vi "FT10_Log TDMS Values.vi"(8 "error in":errorcluster, 9 "Filename Cluster in":T1, 10 "Log Cluster in":T6, 11 "Log Loop Cluster in":T2={"tdms file out"=refnum, "t0"="", "Generator Serial Number in"="T1234567DX"}) -> (0 "error out":errorcluster, 3 "Log Loop Cluster out":T2={"tdms file out"=refnum, "t0"="", "Generator Serial Number in"="T1234567DX"})   [LabVIEW 2024]
doc: "Saves current and diff voltage to the TDMS file created when application started."
uses:
  Controls/Control_Log Cluster.ctl
  Controls/Control_Log Time.ctl
  Controls/Control_Log Waveform Cluster - Current.ctl
  Controls/Control_Log Analysis Cluster - Current.ctl
  Controls/Control_Log Activation Settings Cluster.ctl
  Controls/Control_Log Unitherm Load.ctl
  Controls/Control_Log Port.ctl
  Controls/Control_Log Mode.ctl
  Controls/Control_Log Power Level.ctl
  Controls/Control_Log Waveform Cluster - Diff Voltage.ctl
  Controls/Control_Log Analysis Cluster - Diff Voltage.ctl
  Controls/Control_Log Loop Cluster.ctl
  Controls/Control_Log TDMS Filename.ctl
  Controls/Control_Log t0.ctl
  Controls/Control_Serial Number.ctl
  Controls/Control_Log Filename Cluster.ctl
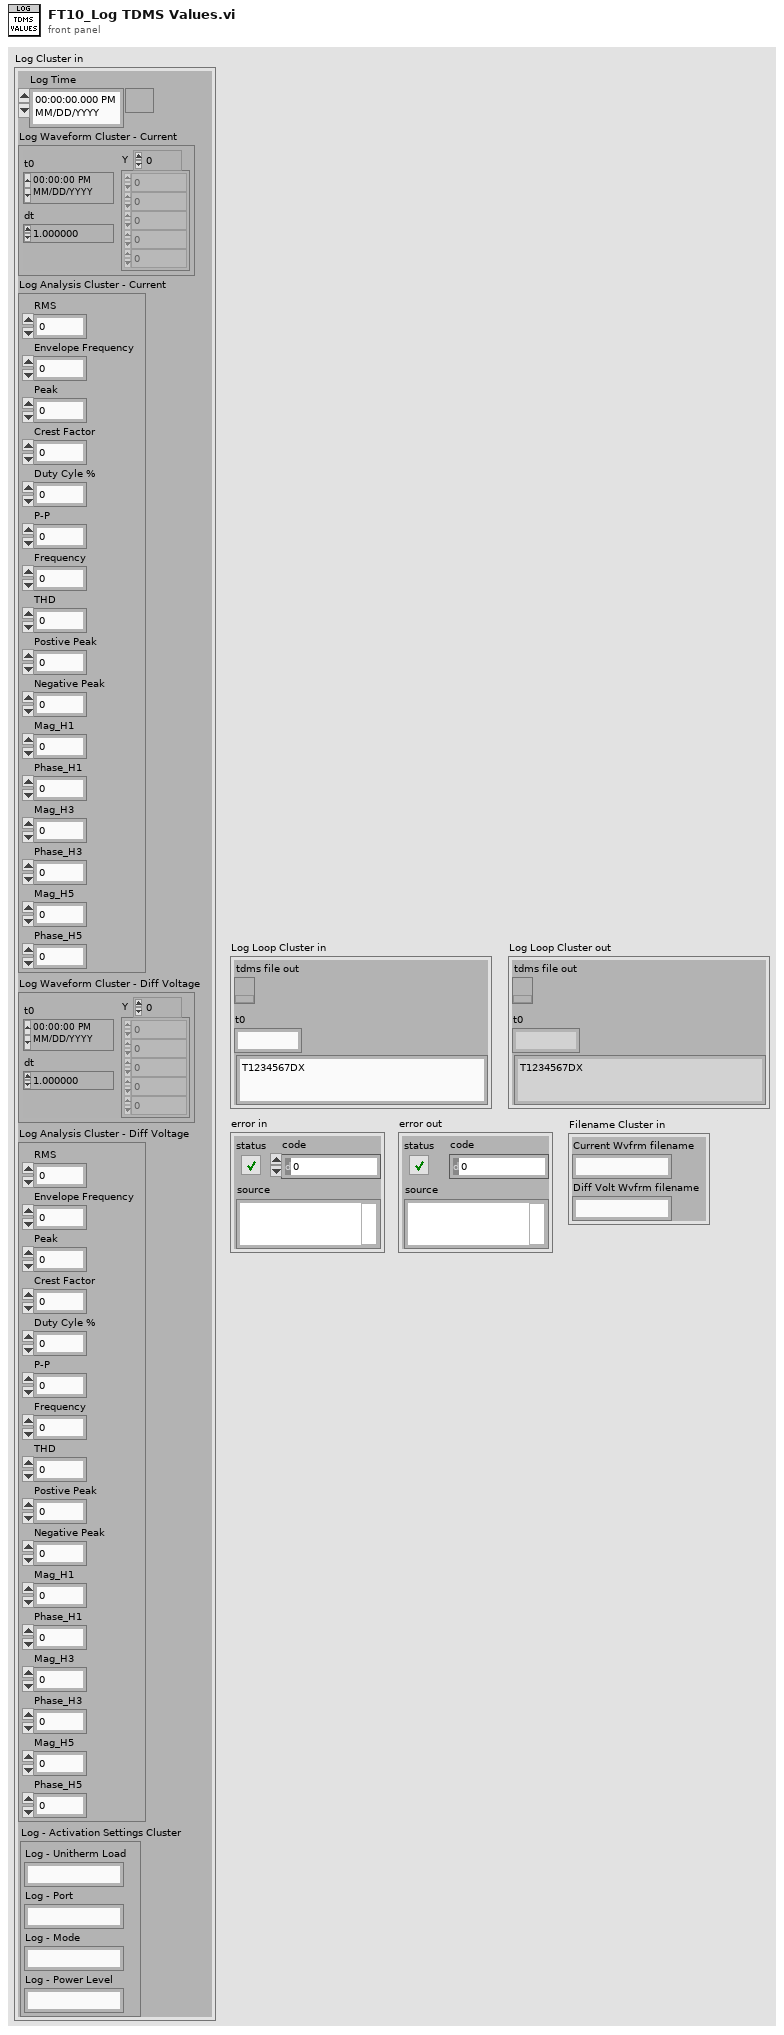
[diagram p1: front panel]
types:
  T1 = typedef "Control_Log Filename Cluster.ctl" = cluster{"Current Wvfrm filename":string, "Diff Volt Wvfrm filename":string}
  T2 = typedef "Control_Log Loop Cluster.ctl" = cluster{"tdms file out":T3, "t0":T4, "Generator Serial Number in":T5}
  T3 = typedef "Control_Log TDMS Filename.ctl" = refnum<k34>
  T4 = typedef "Control_Log t0.ctl" = string
  T5 = typedef "Control_Serial Number.ctl" = string
  T6 = typedef "Control_Log Cluster.ctl" = cluster{"Log Time":T7, "Log Waveform Cluster - Current":T8, "Log Analysis Cluster - Current":T9, "Log - Activation Settings Cluster":T10, "Log Waveform Cluster - Diff Voltage":T15, "Log Analysis Cluster - Diff Voltage":T16}
  T7 = typedef "Control_Log Time.ctl" = timestamp
  T8 = typedef "Control_Log Waveform Cluster - Current.ctl" = waveform(dbl)
  T9 = typedef "Control_Log Analysis Cluster - Current.ctl" = cluster{"RMS":dbl, "Envelope Frequency":dbl, "Peak":dbl, "Crest Factor":dbl, "Duty Cyle %":dbl, "P-P":dbl, "Frequency":dbl, "THD":dbl, "Postive Peak":dbl, "Negative Peak":dbl, "Mag_H1":dbl, "Phase_H1":dbl, "Mag_H3":dbl, "Phase_H3":dbl, "Mag_H5":dbl, "Phase_H5":dbl}
  T10 = typedef "Control_Log Activation Settings Cluster.ctl" = cluster{"Log - Unitherm Load":T11, "Log - Port":T12, "Log - Mode":T13, "Log - Power Level":T14}
  T11 = typedef "Control_Log Unitherm Load.ctl" = string
  T12 = typedef "Control_Log Port.ctl" = string
  T13 = typedef "Control_Log Mode.ctl" = string
  T14 = typedef "Control_Log Power Level.ctl" = string
  T15 = typedef "Control_Log Waveform Cluster - Diff Voltage.ctl" = waveform(dbl)
  T16 = typedef "Control_Log Analysis Cluster - Diff Voltage.ctl" = cluster{"RMS":dbl, "Envelope Frequency":dbl, "Peak":dbl, "Crest Factor":dbl, "Duty Cyle %":dbl, "P-P":dbl, "Frequency":dbl, "THD":dbl, "Postive Peak":dbl, "Negative Peak":dbl, "Mag_H1":dbl, "Phase_H1":dbl, "Mag_H3":dbl, "Phase_H3":dbl, "Mag_H5":dbl, "Phase_H5":dbl}
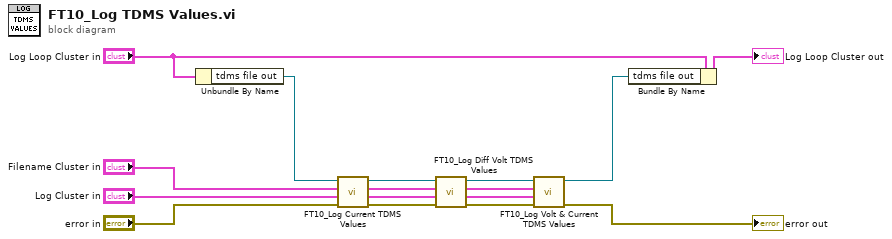
[diagram p0: block diagram]
diagram:
  n1 = Unbundle By Name("Log Loop Cluster in") -> ("tdms file out"=w15:T3)
  n2 = call "FT10_Log Current TDMS Values.vi"("error in (no error)"="error in", "Log Cluster in"="Log Cluster in", "Filename Cluster in"="Filename Cluster in", "Refnum in"=w15) -> ("error out"=w10:errorcluster, "Log Cluster out"=w11:T6, "Filename Cluster out"=w7:T1, "tdms file out"=w14:refnum<k34>)  [unwired: 4 in]
  n3 = call "FT10_Log Diff Volt TDMS Values.vi"("error in (no error)"=w10, "Log Cluster in"=w11, "Filename Cluster in"=w7, "Refnum in"=w14) -> ("error out"=w4:errorcluster, "Log Cluster out"=w1:T6, "Filename Cluster out"=w2:T1, "tdms file out"=w6:refnum<k34>)  [unwired: 4 in]
  n4 = call "FT10_Log Volt & Current TDMS Values.vi"("error in (no error)"=w4, "Log Cluster in"=w1, "Filename Cluster in"=w2, "Refnum in"=w6) -> ("error out"=→"error out":errorcluster, "tdms file out"=w5:refnum<k34>)  [unwired: 4 in, 2 out]
  n5 = Bundle By Name(cluster="Log Loop Cluster in", "tdms file out"=w5) -> (→"Log Loop Cluster out":T2)
